vi "Do.vi"(8 "error in (no error)":errorcluster, 10 "Actor in":refnum<class "Actor.lvclass">, 11 "xps_panel_generate_pvt_trajectory Msg":refnum<class "xps_panel_generate_pvt_trajectory Msg.lvclass">) -> (0 "error out":errorcluster, 2 "Actor out":refnum<class "Actor.lvclass">)   [LabVIEW 2015, in "xps_panel_generate_pvt_trajectory Msg.lvclass"]
doc: "This VI delivers the message to the actor by calling the appropriate method(s) on the actor."
uses:
  xps_panel_generate_pvt_trajectory Msg.lvclass
  <vilib>/ActorFramework/Actor/Actor.lvclass
  xps_panel/newport_xps_panel.lvclass
  xps_panel_generate_pvt_trajectory Msg.lvclass/xps_panel_generate_pvt_trajectory Msg.ctl
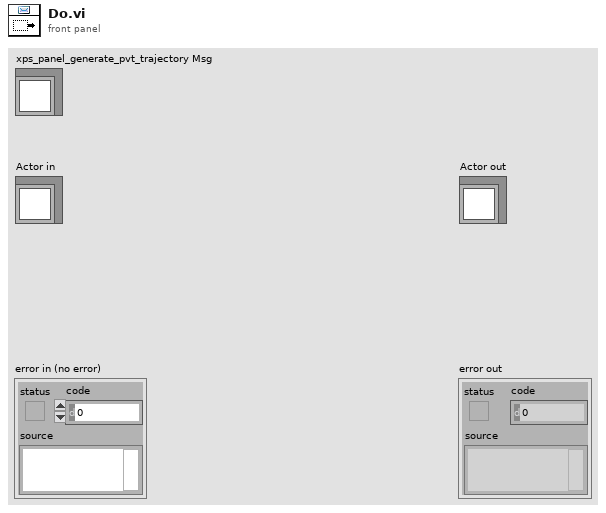
[diagram p1: front panel]
types:
  T1 = typedef "dither_trajectory_settings.ctl" = cluster{"PVT Ampl (nm)":dbl, "Dither Period (s)":dbl, "Type":T2, "Name":string}
  T2 = typedef "dither_trajectory_types.ctl" = enum16{"Sawtooth"}
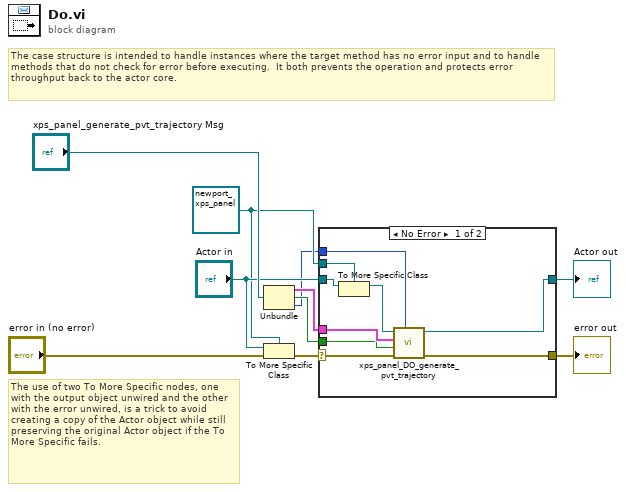
[diagram p0: block diagram]
diagram:
  w4 = refnum<class "newport_xps_panel.lvclass"> refnum ("Actor in")
  # "The use of two To More Specific nodes, one with the output object unwired and the other with the error unwired, is a trick to avoid creating a copy of the Actor object while still preserving the original Actor object if the To More Specific fails."
  # "The case structure is intended to handle instances where the target method has no error input and to handle methods that do not check for error before executing.  It both prevents the operation and protects error throughput back to the actor core."
  n1 = Unbundle("xps_panel_generate_pvt_trajectory Msg") -> (w3:T1, w2:bool, w1:u32)
  n2 = To More Specific Class(target class=w4, reference="Actor in", error in="error in (no error)") -> (error out=w8:errorcluster)  [unwired: 1 out]
  n3 = case shown="No Error" w8 {
    selector: w8 -> [w17 w21]
    tunnel: [w19 w21] -> w7
    tunnel: [w18 w20] -> w6
    tunnel: "Actor in" -> [w16 w20]
    tunnel: w4 -> [w15 _]
    tunnel: w3 -> [w13 _]
    tunnel: w2 -> [w12 _]
    tunnel: w1 -> [w11 _]
    frame No Error {
      n4 = To More Specific Class(target class=w15, reference=w16) -> (specific class reference=w14:refnum<class "newport_xps_panel.lvclass">)  [unwired: 1 in, 1 out]
      n5 = call "xps_panel_DO_generate_pvt_trajectory.vi"("Dither Cycles"=w11, "error in (no error)"=w17, "custom?"=w12, "Custom Dither Trajectory"=w13, "newport_xps_panel in"=w14) -> ("error out"=w19:errorcluster, "newport_xps_panel out"=w18:refnum<class "newport_xps_panel.lvclass">)  [unwired: 5 in]
    }
    frame Error {
      # "If type check fails, pass the original object out again."
    }
  }
  "error out" <- w7
  "Actor out" <- w6
